vi "LuaVIEW Stack to String.vi"(5 "LuaVIEW reference in":T1, 11 "error in (no error)":errorcluster) -> (4 "string":string, 6 "LuaVIEW reference out":T1, 15 "error out":errorcluster)   [LabVIEW 2012]
doc: "Removes the elements present on the stack and converts them into a space-separated string terminated by a linefeed that is suited for printing. This VI is used by print() and similar functions. When converting an element to a string, this function uses the \"tostring\" function, which respects \"__tostring\" metamethods. You can therefore customize the print formatting by overriding \"tostring\" or defining meta methods."
uses:
  typedefs/t_LuaVIEW Reference.ctl
  typedefs/et_LuaVIEW CIN Actions.ctl
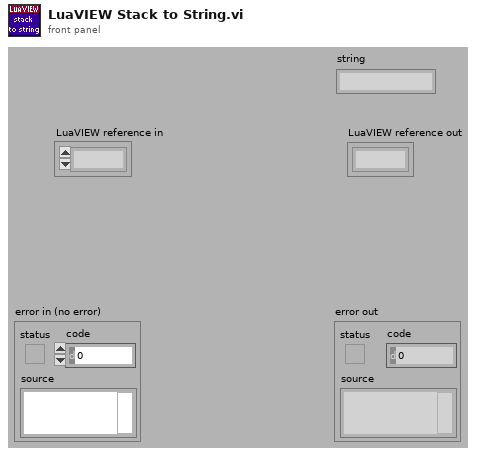
[diagram p1: front panel]
types:
  T1 = typedef "t_LuaVIEW Reference.ctl" = refnum<k1>
  T2 = typedef "et_LuaVIEW CIN Actions.ctl" = enum16{"checksynopsis", "_open", "_registerpublic", "_registerexport", "__never_an_error_result_ns", "luaversion", "cinversion", "_totals", "_taskcount", "pathological", "_unregnextpublic", "registryusecount", "__per_state_actions", "regsetprivate", "regsetindex", "regsetmodule", "_revokeexports", "_usepublic", "prepare", "compile", "execute", "call", "unregstaterefs", "_close", "pullboolean", "pullnumber", "pullI8", "pullU8", "pullI16", "pullU16", "pullI32", "pullU32", "pullobject", "pullrefnum", "pullstring", "pullflat", "pushflat", "pushobject", "getattribute", "setattribute", "stacktostring", "_startyieldtest", "_endyieldtest", "_pollprintbuffer", "__never_an_error_result_ps", "_pollexport", "setclone", "forcecleanup", "gettop", "clearstack", "insert", "pushboolean", "pushnumber", "pushrefnum", "pushstring", "pushnil", "pushvalue", "gettaskref", "settaskref"}
  T3 = typedef "et_LuaVIEW CIN Results.ctl" = enum16{"OK", "error", "main", "call", "clonecall", "modulecall", "exportcall", "index", "yield"}
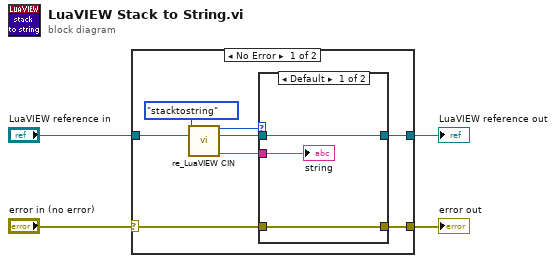
[diagram p0: block diagram]
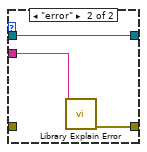
[diagram p2: hidden frame]
diagram:
  n1 = case shown="No Error" "error in (no error)" {
    selector: "error in (no error)" -> [w7 w20]
    tunnel: [w5 w19] -> w4
    tunnel: [w8 w20] -> w3
    tunnel: "LuaVIEW reference in" -> [w11 w19]
    frame No Error {
      n2 = call "re_LuaVIEW CIN.vi"("action"=et_LuaVIEW_CIN_Actions."stacktostring", "LuaVIEW reference in"=w11) -> ("result"=w10:T3, "LuaVIEW reference out"=w6:T1, "string out"=w9:string)  [unwired: 7 in, 4 out]
      n3 = case shown="Default" w10 {
        tunnel: w9 -> [w15 w18]
        tunnel: [w14 w17] -> w8
        tunnel: w7 -> [w14 _]
        tunnel: w6 -> [w13 w16]
        tunnel: [w13 w16] -> w5
        frame Default {
          "string" <- w15
        }
        frame "error" {
          n4 = call "Library Explain Error.vi"("explanation prefix (none)"=w18) -> ("explained error"=w17:errorcluster)  [unwired: 14 in]
        }
      }
    }
    frame Error {
    }
  }
  "LuaVIEW reference out" <- w4
  "error out" <- w3
